vi "Send ADC Command.vi"(8 "error in":errorcluster, 9 "Chanel":u8, 10 "Device":string, 11 "Serial Devices in":refnum<class "Serial Devices.lvclass">) -> (0 "error out":errorcluster, 1 "Expected":string, 2 "Command":string, 3 "Serial Devices out":refnum<class "Serial Devices.lvclass">)   [LabVIEW 2019, in "Serial Devices.lvlib" / "Serial Devices.lvclass"]
uses:
  Serial Devices.lvclass
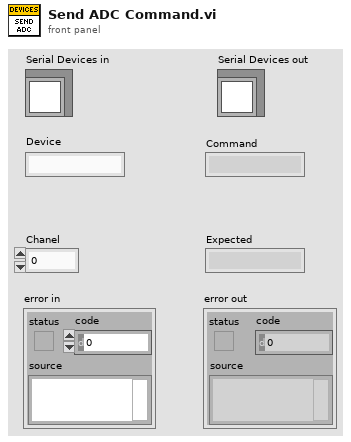
[diagram p1: front panel]
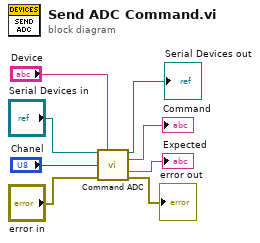
[diagram p0: block diagram]
diagram:
  n1 = call "Command ADC.vi"("Serial Devices in"="Serial Devices in", "Device"="Device", "Chanel"="Chanel", "error in (no error)"="error in") -> ("Serial Devices out"=→"Serial Devices out":refnum<class "Serial Devices.lvclass">, "Command"=→"Command":string, "Expected"=→"Expected":string, "error out"=→"error out":errorcluster)  [unwired: 8 in]
